vi "Untitled 2.vi"() -> ()   [LabVIEW 2020]
panel:
  in  "stop 2":bool
  in  "milliseconds to wait 2":u32
  in  "°F 2":dbl(slide) scale=0.0..10.0
  in  "?":dbl
  in  "Boolean 2":bool
  out "Numeric 2":i32
  out "Thermometer 2":dbl(slide) scale=0.0..100.0 scale format="%#_3g"
  out "Thermometer":dbl(slide) scale=0.0..100.0 scale format="%#_3g"
  out "Numeric":i32
  in  "Boolean":bool
  in  "?":dbl
  in  "°F":dbl(slide) scale=0.0..10.0
  in  "milliseconds to wait":u32
  in  "stop":bool
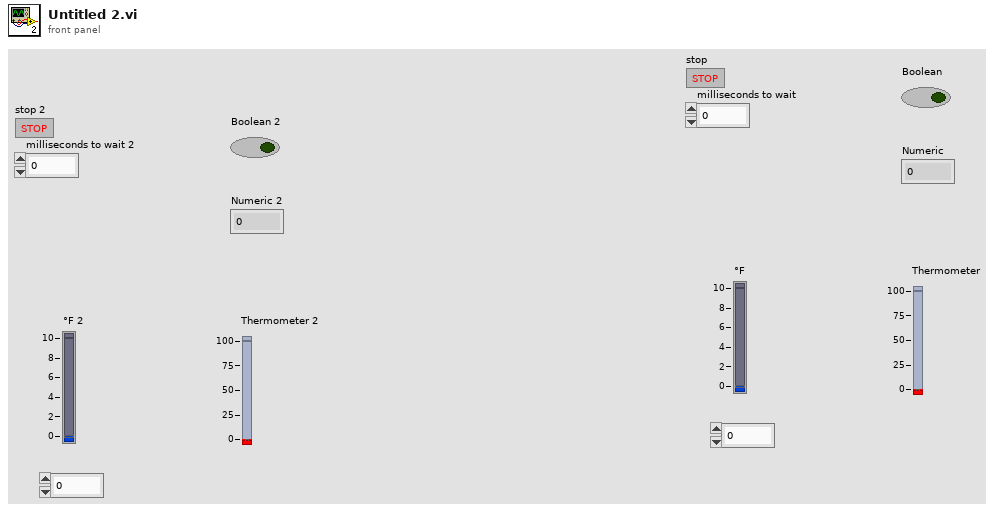
[diagram p1: front panel]
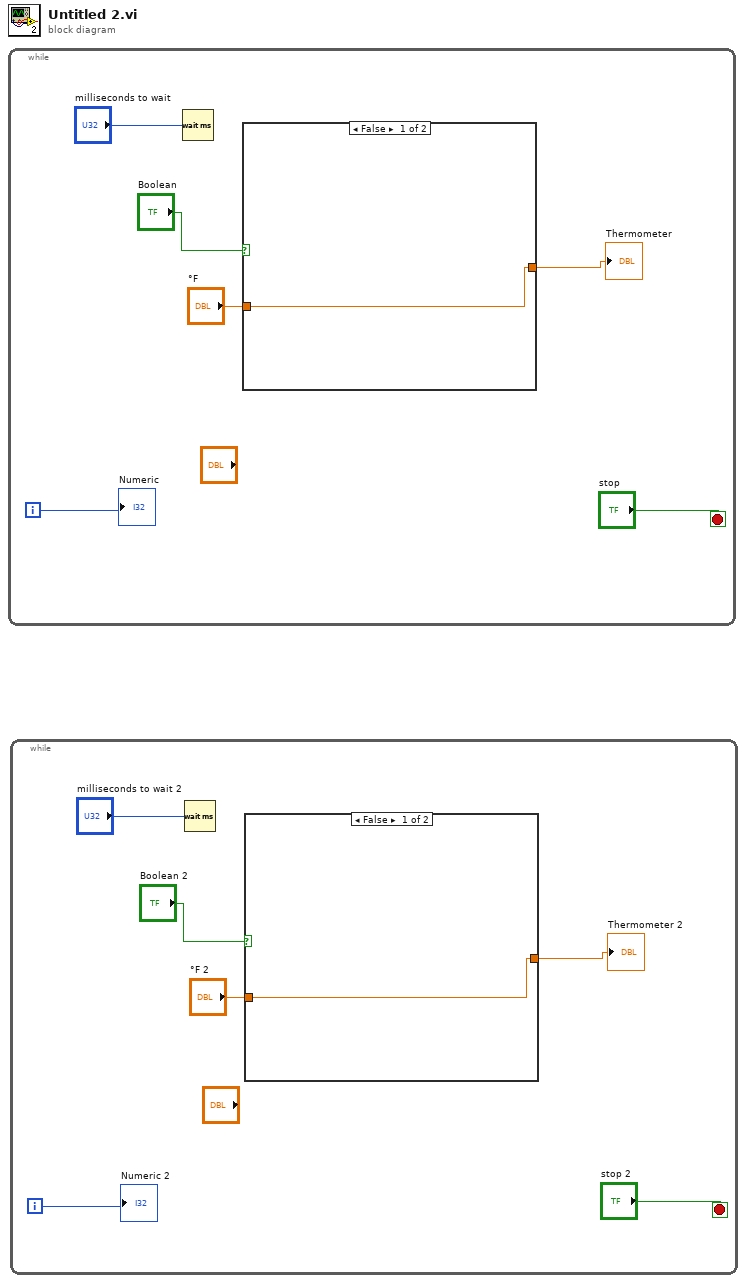
[diagram p0: block diagram]
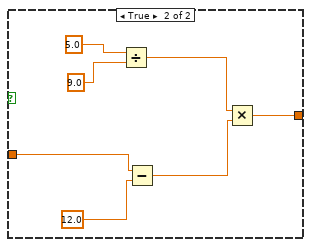
[diagram p2: hidden frame]
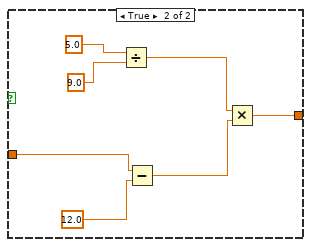
[diagram p3: hidden frame]
diagram:
  n1 = while {
    i -> [w3]
    stop <- "stop" stop-if-true
    n2 = Wait (ms)(milliseconds to wait="milliseconds to wait") -> ()  [unwired: 1 out]
    n3 = case shown="False" "Boolean" {
      tunnel: "°F" -> [w7 w9]
      tunnel: [w7 w8] -> w2
      frame False {
      }
      frame True {
        n4 = Divide(x=5.0, y=9.0 ("x")) -> (x/y=w12:dbl)
        n5 = Subtract(x=w9, y=12.0 ("x")) -> (x-y=w11:dbl)
        n6 = Multiply(x=w12, y=w11) -> (x*y=w8:dbl)
      }
    }
    "Thermometer" <- w2
    "Numeric" <- w3
  }
  n7 = while {
    i -> [w17]
    stop <- "stop 2" stop-if-true
    n8 = Wait (ms)(milliseconds to wait="milliseconds to wait 2") -> ()  [unwired: 1 out]
    n9 = case shown="False" "Boolean 2" {
      tunnel: "°F 2" -> [w21 w23]
      tunnel: [w21 w22] -> w16
      frame False {
      }
      frame True {
        n10 = Divide(x=5.0, y=9.0 ("x")) -> (x/y=w26:dbl)
        n11 = Subtract(x=w23, y=12.0 ("x")) -> (x-y=w25:dbl)
        n12 = Multiply(x=w26, y=w25) -> (x*y=w22:dbl)
      }
    }
    "Thermometer 2" <- w16
    "Numeric 2" <- w17
  }
